vi "Write Fisrt Time Series.vi"(8 "error in (no error)":errorcluster, 10 "Fisrt Time Series":dbl, 11 "Readout Charact in":refnum<class "Readout Charact.lvclass">) -> (0 "error out":errorcluster, 3 "Readout Charact out":refnum<class "Readout Charact.lvclass">)   [LabVIEW 2018, in "Readout Charact.lvclass"]
uses:
  Readout Charact.lvclass
  Readout Charact.lvclass/Readout Charact.ctl
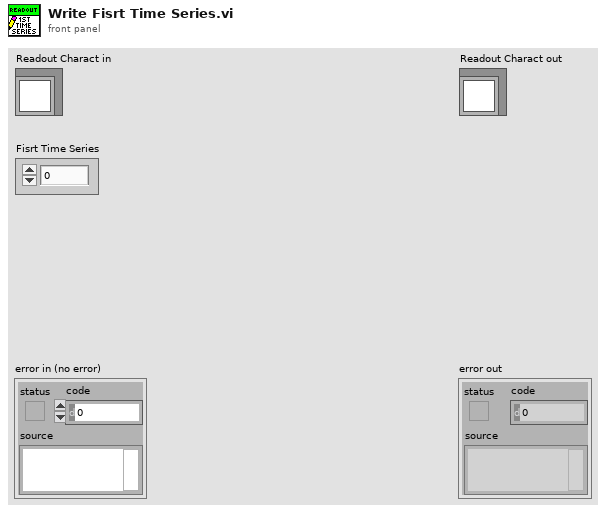
[diagram p1: front panel]
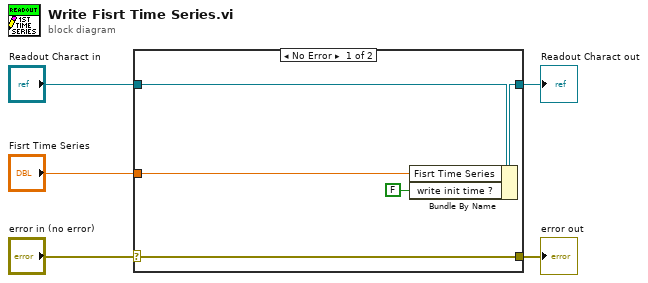
[diagram p0: block diagram]
diagram:
  n1 = case shown="No Error" "error in (no error)" {
    selector: "error in (no error)" -> [w10 w11]
    tunnel: [w10 w11] -> w4
    tunnel: [w8 w12] -> w2
    tunnel: "Readout Charact in" -> [w9 w12]
    tunnel: "Fisrt Time Series" -> [w7 _]
    frame No Error {
      n2 = Bundle By Name(cluster=w9, "Fisrt Time Series"=w7, "write init time ?"=FALSE) -> (w8:refnum<class "Readout Charact.lvclass">)
    }
    frame Error {
    }
  }
  "error out" <- w4
  "Readout Charact out" <- w2
